vi "Measure all.vi"(8 "error in (no error)":errorcluster, 11 "Digital Multimeters in":refnum<class "Digital Multimeter.lvclass">[](array[class])) -> (0 "error out":errorcluster, 2 "Measurements":T1[](array[typedef]), 3 "Digital Multimeters out":refnum<class "Digital Multimeter.lvclass">[](array[class]), 4 "Units":string[](array[string]), 6 "Values":dbl[](array[numeric]))   [LabVIEW 2020, in "Digital Multimeter.lvclass"]
uses:
  Digital Multimeter.lvclass
  XML Handler/Controls/Result Cluster.ctl
  XML Handler/XML Handler.lvclass
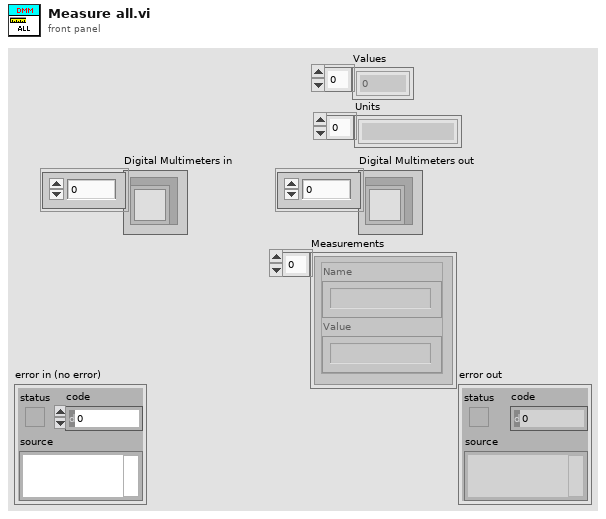
[diagram p1: front panel]
types:
  T1 = typedef "XML Handler.lvclass/Result Cluster.ctl" = cluster{"Name":string, "Value":string}
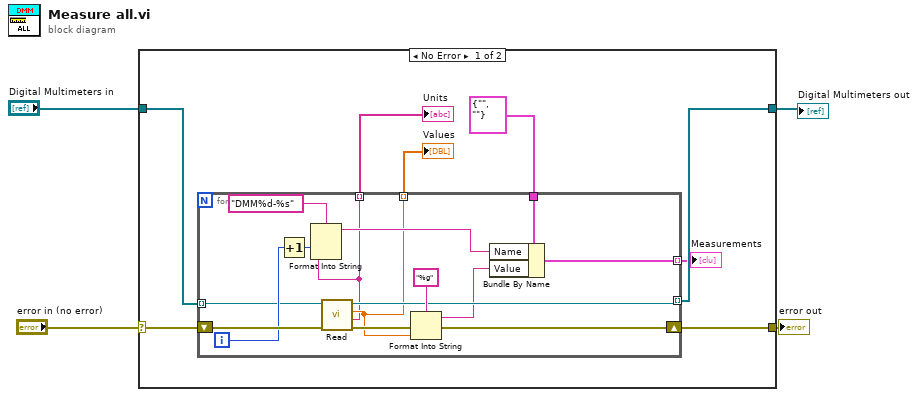
[diagram p0: block diagram]
diagram:
  n1 = case shown="No Error" "error in (no error)" {
    selector: "error in (no error)" -> [w11 w29]
    tunnel: [w12 w29] -> w3
    tunnel: [w9 w28] -> w2
    tunnel: "Digital Multimeters in" -> [w10 w28]
    frame No Error {
      n2 = for {
        tunnel: [w22] -> w9 mode=indexing
        tunnel: T1 {"Name"="", "Value"=""} ("Result Cluster") -> [w24]
        shift-right: [w16] -> w12
        shift-left: w11 -> [w23]
        tunnel: [w18] -> w6 mode=indexing
        tunnel: w10 -> [w15] mode=indexing
        tunnel: [w14] -> w8 mode=indexing
        tunnel: [w13] -> w7 mode=indexing
        i -> [w21]
        n3 = Increment(x=w21) -> (x+1=w20:i32)
        n4 = call-dynamic "Read.vi"("error in (no error)"=w23, "Digital Multimeter in"=w15) -> ("error out"=w17:errorcluster, "Unit"=w13:string, "Measure"=w14:dbl, "Digital Multimeter out"=w22:refnum<class "Digital Multimeter.lvclass">)  [unwired: 5 in, 1 out]
        n5 = Format Into String(format string="DMM%d-%s", w20, w13) -> (resulting string=w25:string)  [unwired: 2 in, 1 out]
        n6 = Format Into String(format string="%g", error in=w17, w14) -> (resulting string=w19:string, error out=w16:errorcluster)  [unwired: 1 in]
        n7 = Bundle By Name(cluster=w24, "Name"=w25, "Value"=w19) -> (w18:T1)
      }
      "Values" <- w8
      "Units" <- w7
      "Measurements" <- w6
    }
    frame Error {
    }
  }
  "error out" <- w3
  "Digital Multimeters out" <- w2
